vi "OpenProjectInCmd.vi"   [LabVIEW 2020]
uses:
  <resource>/dialog/lvconfig.llb/LV Config Read String.vi
types:
  T1 = enum32{"Invalid", "Standard", "Closed", "Hidden", "Minimized", "Maximized"}
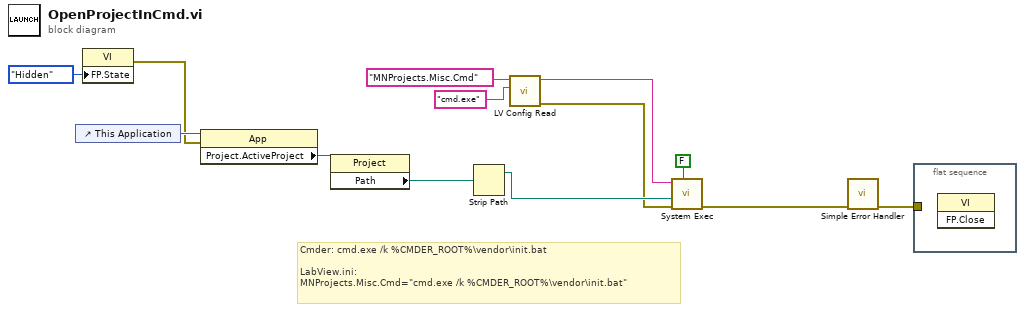
[diagram p0: block diagram]
diagram:
  # "Cmder: cmd.exe /k %CMDER_ROOT%\\vendor\\init.bat\n\nLabView.ini:\nMNProjects.Misc.Cmd=\"cmd.exe /k %CMDER_ROOT%\\vendor\\init.bat\""
  n1 = control-ref of="This Application"() -> (w10:refnum<vi>)
  n2 = property class="VI"("FP.State"=T1."Hidden" ("Front Panel Window:State")) -> (error out=w1:errorcluster)  [unwired: 2 in, 1 out]
  n3 = property class="App"(reference=w10, error in=w1) -> ("Project.ActiveProject"=w9:refnum<vi>)  [unwired: 2 out]
  n4 = property class="Project"(reference=w9) -> ("Path"=w8:path)  [unwired: 1 in, 2 out]
  n5 = Strip Path(path=w8) -> (stripped path=w12:path)  [unwired: 1 out]
  n6 = call-poly <resource>:"LV Config Read.vi"("default value"="cmd.exe" ("command line"), "key"="MNProjects.Misc.Cmd") -> ("error out"=w4:errorcluster, "value"=w5:string)  [unwired: 3 in, 1 out]
  n7 = call <vilib>:"System Exec.vi"("wait until completion? (T)"=FALSE, "error in (no error)"=w4, "working directory"=w12, "command line"=w5) -> ("error out"=w11:errorcluster)  [unwired: 4 in, 3 out]
  n8 = call <vilib>:"Simple Error Handler.vi"("error in (no error)"=w11) -> ("error out"=w3:errorcluster)  [unwired: 4 in, 4 out]
  n9 = flat-sequence {
    tunnel: w3 -> [_]
    frame #0 {
      n10 = invoke class="VI" method="FP.Close"() -> ()  [unwired: 3 in, 3 out]
    }
  }
